vi "JoystickControls.vi"() -> (3 "input cluster 2":T1)   [LabVIEW 2015]
uses:
  Controls.ctl
  References/Refnums.vi
  <vilib>/Rock Robotics/WPI/Utilities/WPI_GetSetVariantRefNum.vi
panel:
  out "input cluster":T1
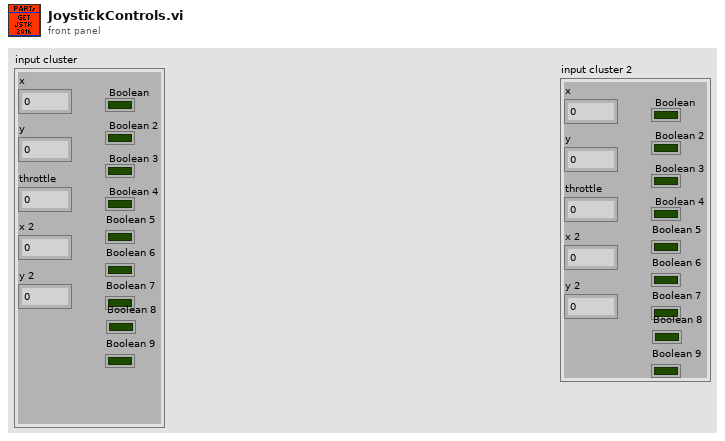
[diagram p1: front panel]
types:
  T1 = typedef "Controls.ctl" = cluster{"x":dbl, "y":dbl, "throttle":dbl, "x 2":dbl, "y 2":dbl, "Boolean":bool, "Boolean 2":bool, "Boolean 3":bool, "Boolean 4":bool, "Boolean 5":bool, "Boolean 6":bool, "Boolean 7":bool, "Boolean 8":bool, "Boolean 9":bool}
  T2 = typedef "WPI_JoystickDevRef.ctl" = cluster{"Device":T3}
  T3 = typedef "WPI_JoystickDeviceEnum.ctl" = enum16{"USB 0", "USB 1", "USB 2", "USB 3", "USB 4", "USB 5"}
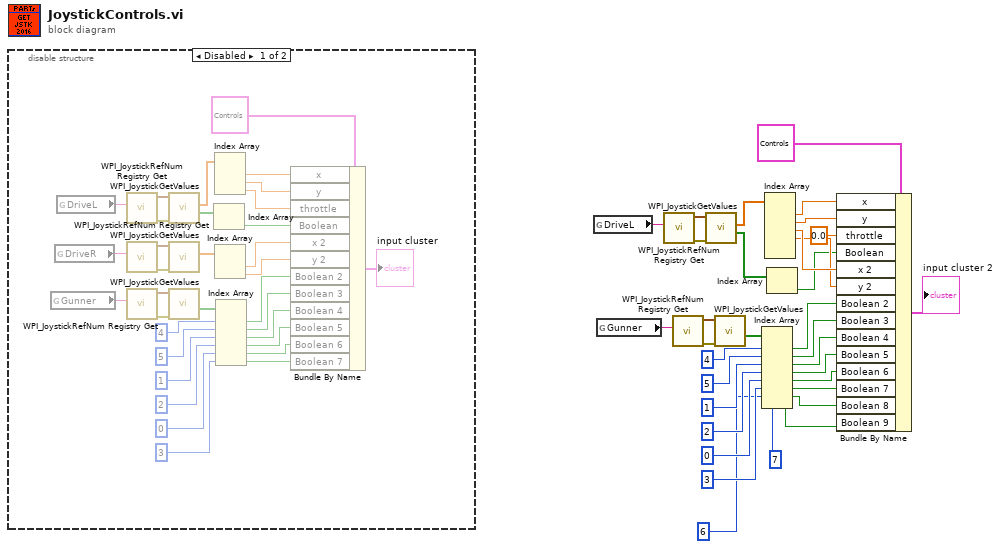
[diagram p0: block diagram]
diagram:
  n1 = disable-structure shown="Disabled" {
    frame Disabled {
      n2 = global read "Refnums.vi" "Gunner"() -> (w47:string)
      n3 = global read "Refnums.vi" "DriveR"() -> (w66:string)
      n4 = global read "Refnums.vi" "DriveL"() -> (w59:string)
      n5 = call <vilib>:"WPI_JoystickRefNum Registry Get.vi"("refnum name"=w59) -> ("error out"=w65:errorcluster, "JoystickDevRef"=w64:T2)  [unwired: 9 in]
      n6 = call <vilib>:"WPI_JoystickRefNum Registry Get.vi"("refnum name"=w66) -> ("error out"=w62:errorcluster, "JoystickDevRef"=w63:T2)  [unwired: 9 in]
      n7 = call <vilib>:"WPI_JoystickRefNum Registry Get.vi"("refnum name"=w47) -> ("error out"=w49:errorcluster, "JoystickDevRef"=w48:T2)  [unwired: 9 in]
      n8 = call <vilib>:"WPI_JoystickGetValues.vi"("error in (no error)"=w65, "JoystickDevRef"=w64) -> ("Buttons"=w54:bool[], "Axes"=w58:dbl[])  [unwired: 5 in, 3 out]
      n9 = call <vilib>:"WPI_JoystickGetValues.vi"("error in (no error)"=w62, "JoystickDevRef"=w63) -> ("Axes"=w52:dbl[])  [unwired: 5 in, 4 out]
      n10 = call <vilib>:"WPI_JoystickGetValues.vi"("error in (no error)"=w49, "JoystickDevRef"=w48) -> ("Buttons"=w46:bool[])  [unwired: 5 in, 4 out]
      n11 = Index Array(array=w54) -> (element=w53:bool)  [unwired: 1 in]
      n12 = Index Array(array=w58) -> (element #1=w57:dbl, element #2=w56:dbl, element #3=w55:dbl)  [unwired: 3 in]
      n13 = Index Array(array=w52) -> (element #1=w51:dbl, element #2=w50:dbl)  [unwired: 2 in]
      n14 = Index Array(array=w46, index #1=4 ("index"), index #2=5 ("index"), index #3=1 ("index"), index #4=2 ("index"), index #5=0 ("index"), index #6=3 ("index")) -> (element #1=w45:bool, element #2=w44:bool, element #3=w43:bool, element #4=w42:bool, element #5=w41:bool, element #6=w40:bool)
      n15 = Bundle By Name(cluster=T1 {"x"=0.0, "y"=0.0, "throttle"=0.0, "x 2"=0.0, "y 2"=0.0, "Boolean"=FALSE, "Boolean 2"=FALSE, "Boolean 3"=FALSE, "Boolean 4"=FALSE, "Boolean 5"=FALSE, "Boolean 6"=FALSE, "Boolean 7"=FALSE, "Boolean 8"=FALSE, "Boolean 9"=FALSE} ("input cluster"), "x"=w57, "y"=w56, "throttle"=w55, "Boolean"=w53, "x 2"=w51, "y 2"=w50, "Boolean 2"=w45, "Boolean 3"=w44, "Boolean 4"=w43, "Boolean 5"=w42, "Boolean 6"=w41, "Boolean 7"=w40) -> (→"input cluster":T1)
    }
    frame Enabled {
    }
  }
  n16 = global read "Refnums.vi" "DriveL"() -> (w15:string)
  n17 = global read "Refnums.vi" "Gunner"() -> (w20:string)
  n18 = call <vilib>:"WPI_JoystickRefNum Registry Get.vi"("refnum name"=w15) -> ("error out"=w13:errorcluster, "JoystickDevRef"=w14:T2)  [unwired: 9 in]
  n19 = call <vilib>:"WPI_JoystickRefNum Registry Get.vi"("refnum name"=w20) -> ("error out"=w18:errorcluster, "JoystickDevRef"=w19:T2)  [unwired: 9 in]
  n20 = call <vilib>:"WPI_JoystickGetValues.vi"("error in (no error)"=w13, "JoystickDevRef"=w14) -> ("Buttons"=w7:bool[], "Axes"=w12:dbl[])  [unwired: 5 in, 3 out]
  n21 = call <vilib>:"WPI_JoystickGetValues.vi"("error in (no error)"=w18, "JoystickDevRef"=w19) -> ("Buttons"=w21:bool[])  [unwired: 5 in, 4 out]
  n22 = Index Array(array=w21, index #1=4 ("index"), index #2=5 ("index"), index #3=1 ("index"), index #4=2 ("index"), index #5=0 ("index"), index #6=3 ("index"), index #7=6 ("index"), index #8=7 ("index")) -> (element #1=w22:bool, element #2=w23:bool, element #3=w24:bool, element #4=w25:bool, element #5=w26:bool, element #6=w27:bool, element #7=w3:bool, element #8=w2:bool)
  n23 = Index Array(array=w12) -> (element #1=w11:dbl, element #2=w10:dbl, element #3=w9:dbl, element #4=w8:dbl)  [unwired: 6 in, 2 out]
  n24 = Index Array(array=w7) -> (element=w6:bool)  [unwired: 1 in]
  n25 = Bundle By Name(cluster=T1 {"x"=0.0, "y"=0.0, "throttle"=0.0, "x 2"=0.0, "y 2"=0.0, "Boolean"=FALSE, "Boolean 2"=FALSE, "Boolean 3"=FALSE, "Boolean 4"=FALSE, "Boolean 5"=FALSE, "Boolean 6"=FALSE, "Boolean 7"=FALSE, "Boolean 8"=FALSE, "Boolean 9"=FALSE} ("input cluster"), "x"=w11, "y"=w10, "throttle"=0.0, "Boolean"=w6, "x 2"=w9, "y 2"=w8, "Boolean 2"=w22, "Boolean 3"=w23, "Boolean 4"=w24, "Boolean 5"=w25, "Boolean 6"=w26, "Boolean 7"=w27, "Boolean 8"=w3, "Boolean 9"=w2) -> (→"input cluster 2":T1)
